vi "Filter Request.vi"(8 "error in (no error)":errorcluster, 10 "request":refnum<class "request.lvclass">, 11 "output_actor in":refnum<class "Output Actor.lvclass">) -> (0 "error out":errorcluster, 1 "Filtered":bool, 2 "request out":refnum<class "request.lvclass">, 3 "output_actor out":refnum<class "Output Actor.lvclass">)   [LabVIEW 2015, in "Output Actor.lvclass"]
uses:
  Output Actor.lvclass
  Request/request.lvclass
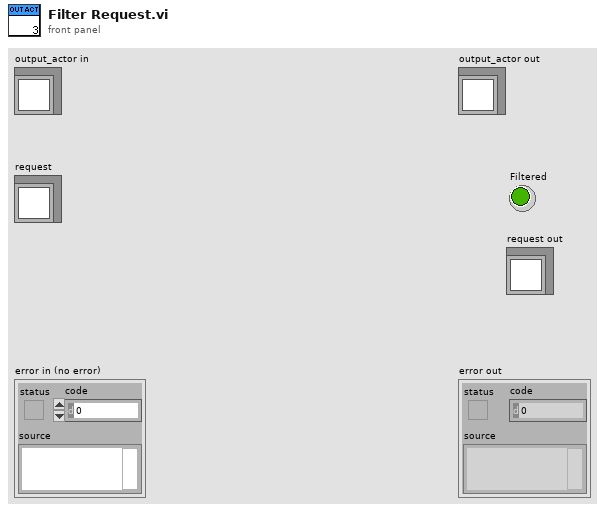
[diagram p1: front panel]
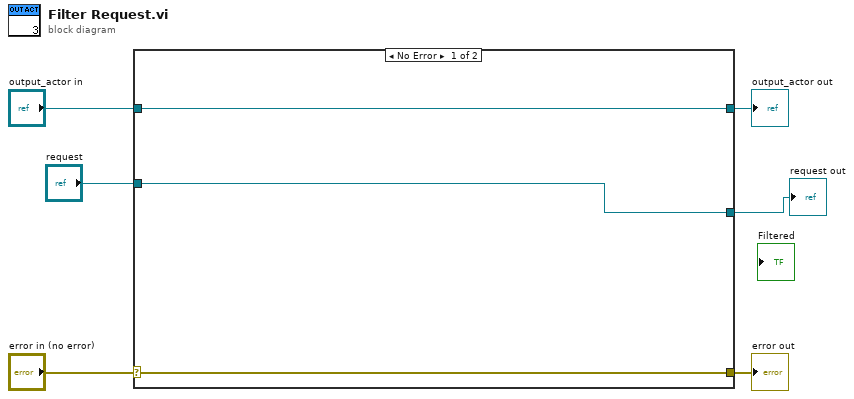
[diagram p0: block diagram]
diagram:
  n1 = case shown="No Error" "error in (no error)" {
    selector: "error in (no error)" -> [w8 w11]
    tunnel: [w8 w11] -> w5
    tunnel: [w9 w10] -> w3
    tunnel: "output_actor in" -> [w9 w10]
    tunnel: [w7 _] -> w2
    tunnel: "request" -> [w7 _]
    frame No Error {
    }
    frame Error {
    }
  }
  "error out" <- w5
  "output_actor out" <- w3
  "request out" <- w2
